vi "Receive Config Data MHLC.vi"(8 "error in (no error)":errorcluster, 10 "Data":variant, 11 "AppMgr in":refnum<class "Application Manager.lvclass">) -> (0 "error out":errorcluster, 3 "AppMgr out":refnum<class "Application Manager.lvclass">)   [LabVIEW 2017, in "Application Manager.lvclass"]
doc: "Receive the startup configuration for the Application Manager and apply these values to the various FP elements, etc."
uses:
  Application Manager.lvclass
  rqp_Receive Config Data.ctl
  <vilib>/Utility/miscctls.llb/LVRectTypeDef.ctl
  Application Manager.lvclass/Application Manager.ctl
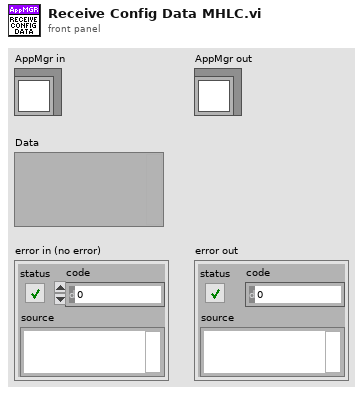
[diagram p1: front panel]
types:
  T1 = typedef "Application Manager.lvclass/rqp_Receive Config Data.ctl" = cluster{"Server Port":u16, "WinBounds":T2, "FP.State":enum32{"Invalid", "Standard", "Closed", "Hidden", "Minimized", "Maximized"}, "Monitor":u16, "Column Widths":u32[]}
  T2 = typedef "LVRectTypeDef.ctl" = cluster{"Left":i16, "Top":i16, "Right":i16, "Bottom":i16}
  T3 = enum32{"Invalid", "Standard", "Closed", "Hidden", "Minimized", "Maximized"}
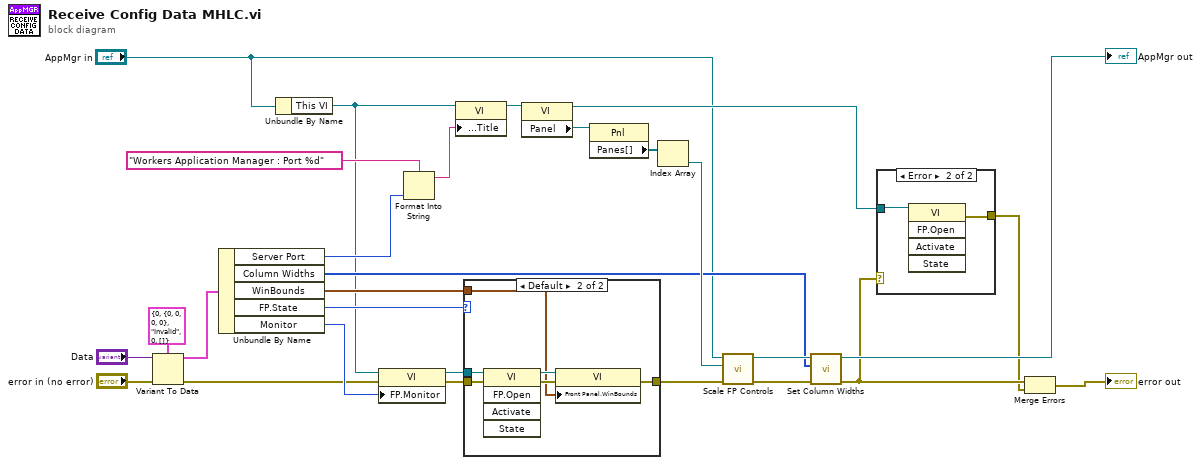
[diagram p0: block diagram]
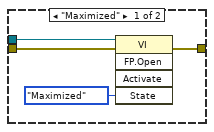
[diagram p3: hidden frame]
diagram:
  n1 = Variant To Data(error in="error in (no error)", type=T1 {"Server Port"=0, "WinBounds"={"Left"=0, "Top"=0, "Right"=0, "Bottom"=0}, "FP.State"=enum."Invalid", "Monitor"=0, "Column Widths"=[]} ("Data"), Variant="Data") -> (data=w14:T1, error out=w1:errorcluster)
  n2 = Unbundle By Name(w14) -> ("Server Port"=w27:u16, "Column Widths"=w10:u32[], "WinBounds"=w22:T2, "FP.State"=w23:T3, "Monitor"=w21:u16)
  n3 = Unbundle By Name("AppMgr in") -> ("This VI"=w8:refnum<vi>)
  n4 = property class="VI"(reference=w8, error in=w1, "FP.Monitor"=w21) -> (reference out=w20:refnum<vi>, error out=w19:errorcluster)
  n5 = Format Into String(format string="Workers Application Manager : Port %d", w27) -> (resulting string=w28:string)  [unwired: 2 in, 1 out]
  n6 = property class="VI"(reference=w8, "Front Panel.Title"=w28) -> (reference out=w9:refnum<vi>)  [unwired: 1 in, 1 out]
  n7 = case shown="Default" w23 {
    tunnel: [w32 w38] -> w24
    tunnel: w19 -> [w31 w37]
    tunnel: w20 -> [w30 w35]
    tunnel: w22 -> [_ w33]
    frame "Maximized" {
      n8 = invoke class="VI" method="FP.Open"(reference=w30, error in=w31, "State"=T3."Maximized" ("Front Panel Window:State")) -> (error out=w32:errorcluster)  [unwired: 2 in, 4 out]
    }
    frame Default {
      n9 = invoke class="VI" method="FP.Open"(reference=w35, error in=w37) -> (reference out=w34:refnum<vi>, error out=w36:errorcluster)  [unwired: 3 in, 3 out]
      n10 = property class="VI"(reference=w34, error in=w36, "Front Panel.WinBounds"=w33) -> (error out=w38:errorcluster)  [unwired: 1 out]
    }
  }
  n11 = property class="VI"(reference=w9) -> (reference out=w6:refnum<vi>, "Panel"=w18:refnum<vi>)  [unwired: 1 in, 1 out]
  n12 = property class="Pnl"(reference=w18) -> ("Panes[]"=w17:refnum<vi>[])  [unwired: 1 in, 2 out]
  n13 = Index Array(array=w17) -> (element=w16:refnum<vi>)  [unwired: 1 in]
  n14 = call "Scale FP Controls.vi"("error in (no error)"=w24, "Pane"=w16, "AppMgr in"="AppMgr in") -> ("error out"=w25:errorcluster, "AppMgr out"=w12:refnum<class "Application Manager.lvclass">)  [unwired: 7 in]
  n15 = call "Set Column Widths.vi"("error in (no error)"=w25, "Column Widths"=w10, "AppMgr in"=w12) -> ("error out"=w7:errorcluster, "AppMgr out"=→"AppMgr out":refnum<class "Application Manager.lvclass">)  [unwired: 7 in]
  n16 = case shown="Error" w7 {
    selector: w7 -> [w39 _]
    tunnel: [w39 w41] -> w4
    tunnel: w6 -> [_ w40]
    frame No Error {
    }
    frame Error {
      n17 = invoke class="VI" method="FP.Open"(reference=w40) -> (error out=w41:errorcluster)  [unwired: 4 in, 4 out]
    }
  }
  n18 = Merge Errors(w7, w4) -> (→"error out":errorcluster)
